vi "ScaleSensorSubVI.vi"(11 "Numeric in":i32) -> (3 "Numeric out":dbl)   [LabVIEW 2021]
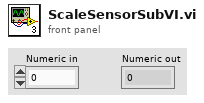
[diagram p1: front panel]
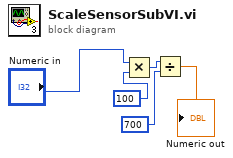
[diagram p0: block diagram]
diagram:
  n1 = Multiply(x="Numeric in", y=100 ("value")) -> (x*y=w2:i32)
  n2 = Divide(x=w2, y=700 ("value")) -> (x/y=→"Numeric out":dbl)
